vi "RSZVB Set NWA Application Priority.vi"(8 "error in (no error)":errorcluster {"code" format="%.0x"}, 9 "Priority (Normal)":i32(ring) items=["Normal", "Above Normal", "High"], 11 "VISA session":refnum<visa-resource-name>) -> (0 "error out":errorcluster {"code" format="%.0x"}, 3 "dup VISA session":refnum<visa-resource-name>)   [LabVIEW 2011]
doc: "Selects the priority of the running NWA application.\n\nRemote-control command(s):\nSYSTem:PRIority NORMal | ANORmal | HIGH"
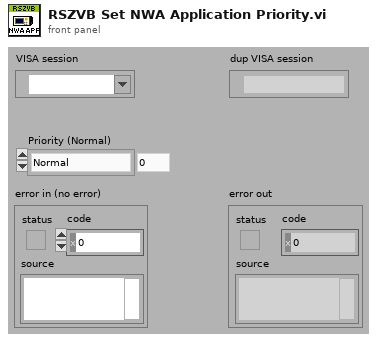
[diagram p1: front panel]
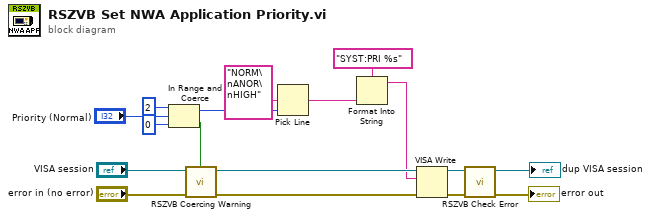
[diagram p0: block diagram]
diagram:
  n1 = In Range and Coerce(upper limit=2 ("lower limit"), x="Priority (Normal)", lower limit=0) -> (coerced(x)=w9:i32, In Range?=w12:bool)
  n2 = call "RSZVB Coercing Warning.vi"("In Range?"=w12, "error in (no error)"="error in (no error)", "VISA session"="VISA session") -> ("error out"=w5:errorcluster, "dup VISA session"=w6:refnum<visa-resource-name>)  [unwired: 7 in]
  n3 = Pick Line(multi-line string="NORM\nANOR\nHIGH", line index=w9) -> (output string=w13:string)  [unwired: 1 in]
  n4 = Format Into String(format string="SYST:PRI %s", w13) -> (resulting string=w2:string)  [unwired: 2 in, 1 out]
  n5 = VISA Write(VISA resource name=w6, write buffer=w2, error in (no error)=w5) -> (VISA resource name out=w14:refnum<visa-resource-name>, error out=w15:errorcluster)  [unwired: 1 out]
  n6 = call "RSZVB Check Error.vi"("error in (no error)"=w15, "VISA session"=w14) -> ("error out"=→"error out":errorcluster, "dup VISA session"=→"dup VISA session":refnum<visa-resource-name>)  [unwired: 8 in]
